vi "CheckChecksum.vi"(11 "String":string) -> (3 "x = y?":bool)   [LabVIEW 2015]
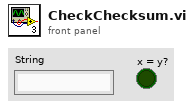
[diagram p1: front panel]
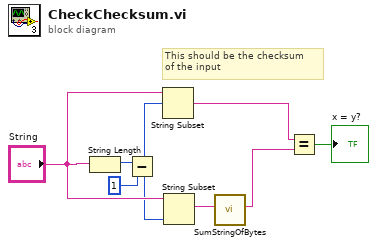
[diagram p0: block diagram]
diagram:
  # "This should be the checksum \nof the input"
  n1 = String Length(string="String") -> (length=w6:i32)
  n2 = Subtract(x=w6, y=1) -> (x-y=w7:i32)
  n3 = String Subset(string="String", offset (0)=w7) -> (substring=w3:string)  [unwired: 1 in]
  n4 = String Subset(string="String", length (rest)=w7) -> (substring=w4:string)  [unwired: 1 in]
  n5 = call "SumStringOfBytes.vi"("String Of Bytes"=w4) -> ("SumAsString"=w2:string)  [unwired: 10 in]
  n6 = Equal?(x=w3, y=w2) -> (x = y?=→"x = y?":bool)
